vi "Generate Path.vi"(11 "User Interface Cluster":T1 {"Serial Settings"."flow control" items=["None"=0, "XON/XOFF"=1, "RTS/CTS"=2, "DTR/DSR"=4]; "Serial Settings"."stop bits" items=["1.0"=10, "1.5"=15, "2.0"=20]; "Serial Settings"."data bits" min=5 max=8 step=1; "Serial Settings"."baud rate" items=["75"=75, "110"=110, "134"=134, "150"=150, "300"=300, "600"=600, "1200"=1200, "1800"=1800, "2400"=2400, "4800"=4800, "7200"=7200, "9600"=9600, "14400"=14400, "19200"=19200, "28800"=28800, "38400"=38400, "56000"=56000, "57600"=57600, "115200"=115200, "128000"=128000, "230400"=230400]}) -> (3 "appended path":path)   [LabVIEW 2019]
uses:
  Controls/User Interface Cluster.ctl
  Serial Comms/Serial - Settings.ctl
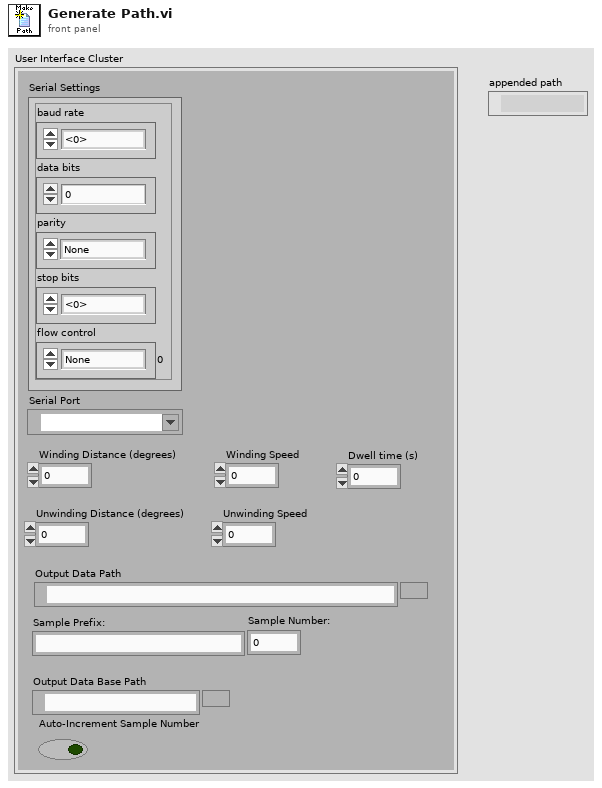
[diagram p1: front panel]
types:
  T1 = typedef "User Interface Cluster.ctl" = cluster{"Serial Settings":T2, "Serial Port":refnum<visa-resource-name>, "Winding Distance (degrees)":dbl, "Winding Speed":dbl, "Dwell time (s)":dbl, "Unwinding Distance (degrees)":dbl, "Unwinding Speed":dbl, "Output Data Path":path, "Sample Prefix:":string, "Sample Number:":u32, "Output Data Base Path":path, "Auto-Increment Sample Number":bool}
  T2 = typedef "Serial - Settings.ctl" = cluster{"baud rate":u32, "data bits":u16, "parity":enum16{"None", "Odd", "Even", "Mark", "Space"}, "stop bits":u16, "flow control":u16}
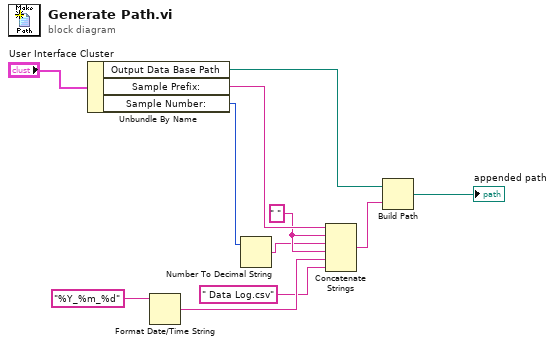
[diagram p0: block diagram]
diagram:
  w6 = " " ("string")
  n1 = Unbundle By Name("User Interface Cluster") -> ("Output Data Base Path"=w9:path, "Sample Prefix:"=w10:string, "Sample Number:"=w11:u32)
  n2 = Format Date/Time String(time format string (%c)="%Y_%m_%d") -> (date/time string=w5:string)  [unwired: 2 in]
  n3 = Number To Decimal String(number=w11) -> (decimal integer string=w1:string)  [unwired: 1 in]
  n4 = Concatenate Strings(w10, w6, w1, w6, w5, " Data Log.csv" ("string")) -> (w2:string)
  n5 = Build Path(base path=w9, name or relative path=w2) -> (appended path=→"appended path":path)
